vi "I2C Grove 8x8 RGB Matrix LED Examples.vi"() -> ()   [LabVIEW 2020, in "CTI-Scratchpad.lvlib"]
uses:
  CTI-Scratchpad.lvlib
  CTI/Identity.ctl
  CTI-Peripheral/RGB LED Matrix/Grove 2 RGB LED Matrix/Data Types/Colors.ctl
  CTI-Peripheral/RGB LED Matrix/Grove 2 RGB LED Matrix/Data Types/Emojis.ctl
  CTI-Peripheral/RGB LED Matrix/Grove 2 RGB LED Matrix/Data Types/Animations.ctl
  CTI/Error Reporting.ctl
  CTI/GPIO Number.ctl
  CTI/I2C Number.ctl
  CTI/Session/Session.lvclass
  CTI-Peripheral/RGB LED Matrix/Grove 2 RGB LED Matrix/Grove 2 RGB LED Matrix.lvclass
  CTI/VisaComms/VisaComms.lvclass
  CTI/CTI.lvlib
panel:
  in  "Animation":T1
  in  "Set Animation":bool
  in  "Emoji":T2 items=["smile", "laugh", "sad", "mad", "angry", "cry", "greedy", "cool", "shy", "awkward", "heart", "small heart", "broken heart", "waterdrop", "flame", "creeper", "mad creeper", "sword", "wooden sword", "crystal sword", "house", "tree", "flower", "umbrella", "rain", "monster", "crab", "duck", "rabbit", "cat", "up", "down", "left", "right", "smiley face"]
  in  "Set Emoji":bool
  in  "String":string
  in  "Set String":bool
  in  "Colour":T3 items=["red"=0, "orange"=18, "yellow"=24, "green"=82, "cyan"=127, "blue"=170, "purple"=195, "pink"=220, "white"=254, "black"=255]
  in  "Number":u16 max=9 step=1
  out "Version":string
  in  "Set Number":bool
  out "Identity":T4
  in  "stop":bool
  in  "Grove Connector":enum16{"I2C0", "I2C1"}(ring)
  out "error out":errorcluster
  in  "Port":refnum<visa-resource-name>="COM4"
  # "https://wiki.seeedstudio.com/Grove-RGB_LED_Matrix_w-Driver/"
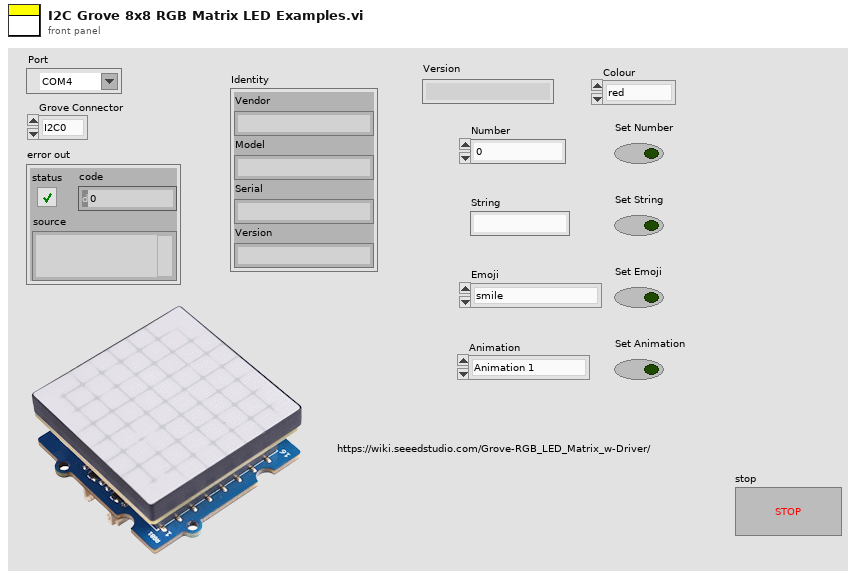
[diagram p1: front panel]
types:
  T1 = typedef "CTI-Peripheral.lvlib/Grove 2 RGB LED Matrix.lvclass/Animations.ctl" = enum16{"Animation 1", "Animation 2", "Rainbow Cycle", "Fire", "Walking", "Broken Heart"}
  T2 = typedef "CTI-Peripheral.lvlib/Grove 2 RGB LED Matrix.lvclass/Emojis.ctl" = u16
  T3 = typedef "CTI-Peripheral.lvlib/Grove 2 RGB LED Matrix.lvclass/Colors.ctl" = u8
  T4 = typedef "CTI.lvlib/Identity.ctl" = cluster{"Vendor":string, "Model":string, "Serial":string, "Version":string}
  T5 = typedef "CTI.lvlib/Error Reporting.ctl" = enum16{"Minimal", "Moderate", "Full"}
  T6 = typedef "CTI.lvlib/I2C Number.ctl" = i8
  T7 = typedef "CTI.lvlib/GPIO Number.ctl" = i8
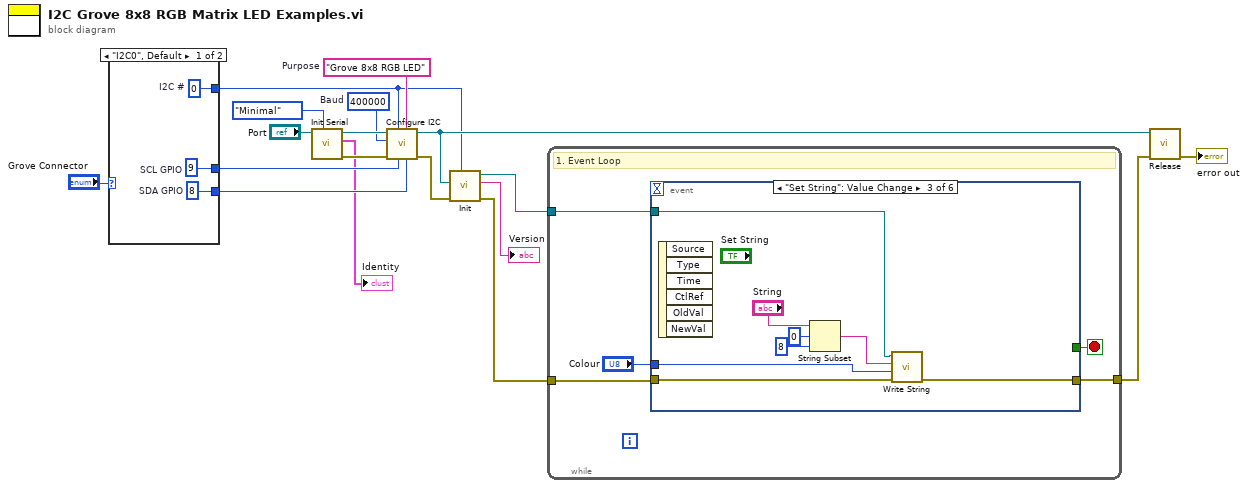
[diagram p0: block diagram]
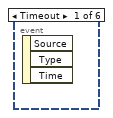
[diagram p2: hidden frame]
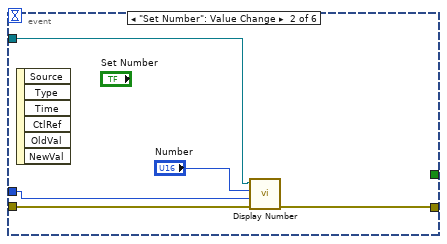
[diagram p3: hidden frame]
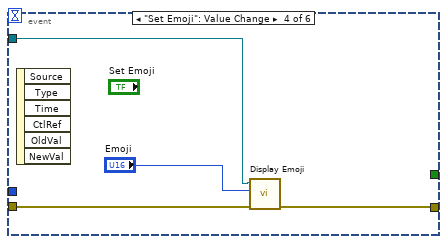
[diagram p4: hidden frame]
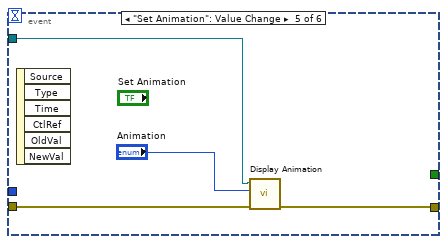
[diagram p5: hidden frame]
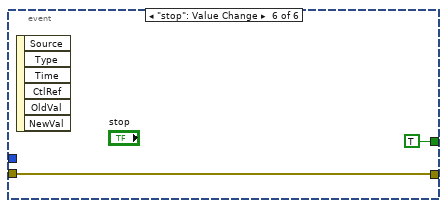
[diagram p6: hidden frame]
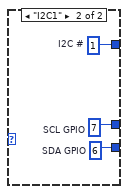
[diagram p7: hidden frame]
diagram:
  w13 = "Grove 8x8 RGB LED"  # Purpose
  w14 = u32 400000  # Baud
  n1 = case shown="\"I2C0\", Default" "Grove Connector" {
    tunnel: [w21 w24] -> w9
    tunnel: [w20 w23] -> w8
    tunnel: [w19 w22] -> w7
    frame "I2C0", Default {
      w19 = T6 0  # I2C #
      w20 = T7 8  # SDA GPIO
      w21 = T7 9  # SCL GPIO
    }
    frame "I2C1" {
      w22 = T6 1  # I2C #
      w23 = T7 6  # SDA GPIO
      w24 = T7 7  # SCL GPIO
    }
  }
  n2 = call "Init Serial.vi"("Error Checking (Full)"=Error_Reporting."Minimal", "VISA resource name in"="Port") -> ("error out"=w15:errorcluster, "Identity"=→"Identity":T4, "Session"=w16:refnum<class "Session.lvclass">)  [unwired: 7 in]
  n3 = call "Configure I2C.vi"("SDA GPIO"=w8, "Purpose (\"I2C\")"=w13, "SCL GPIO"=w9, "I2C #"=w7, "error in (no error)"=w15, "Baud"=w14, "Session in"=w16) -> ("error out"=w12:errorcluster, "Session out"=w11:refnum<class "Session.lvclass">)  [unwired: 3 in]
  n4 = call "Init.vi"("I2C #"=w7, "error in (no error)"=w12, "Session In"=w11) -> ("error out"=w5:errorcluster, "Version"=→"Version":string, "Grove 2 RGB LED Matrix Out"=w2:refnum<class "Grove 2 RGB LED Matrix.lvclass">)  [unwired: 6 in]
  n5 = while {
    tunnel: w5 -> [w28]
    tunnel: [w27] -> w4
    tunnel: w2 -> [w29]
    stop <- w26 stop-if-true
    # "1. Event Loop"
    n6 = event shown="[2] \"Set String\": Value Change" {
      selector: _ -> [_ _ _ _ _ _]
      dyn-events: _ -> [_ _ _ _ _ _]
      timeout: _ -> [_ _ _ _ _ _]
      tunnel: w29 -> [_ w32 w40 w44 w48 _]
      tunnel: w28 -> [_ w34 w42 w46 w50 w52]
      tunnel: [_ w33 w41 w45 w49 w52] -> w27
      tunnel: [_ _ _ _ _ TRUE] -> w26
      tunnel: "Colour" -> [_ w30 w39 _ _ _]
      event Timeout {
        n7 = event-data() -> ()  [unwired: 1 in, 3 out]
      }
      event "Set Number": Value Change {
        n8 = event-data() -> ()  [unwired: 1 in, 6 out]
        n9 = call-dynamic "Display Number.vi"("error in (no error)"=w34, "Colour"=w30, "Numeric"="Number", "Grove 2 RGB LED Matrix In"=w32) -> ("error out"=w33:errorcluster)  [unwired: 6 in, 1 out]
      }
      event "Set String": Value Change {
        n10 = event-data() -> ()  [unwired: 1 in, 6 out]
        n11 = String Subset(string="String", offset (0)=0, length (rest)=8 ("length (rest)")) -> (substring=w35:string)
        n12 = call-dynamic "Write String.vi"("error in (no error)"=w42, "Colour"=w39, "String"=w35, "Grove 2 RGB LED Matrix In"=w40) -> ("error out"=w41:errorcluster)  [unwired: 6 in, 1 out]
      }
      event "Set Emoji": Value Change {
        n13 = event-data() -> ()  [unwired: 1 in, 6 out]
        n14 = call-dynamic "Display Emoji.vi"("error in (no error)"=w46, "Emoji"="Emoji", "Grove 2 RGB LED Matrix In"=w44) -> ("error out"=w45:errorcluster)  [unwired: 7 in, 1 out]
      }
      event "Set Animation": Value Change {
        n15 = event-data() -> ()  [unwired: 1 in, 6 out]
        n16 = call-dynamic "Display Animation.vi"("error in (no error)"=w50, "Animations"="Animation", "Grove 2 RGB LED Matrix In"=w48) -> ("error out"=w49:errorcluster)  [unwired: 7 in, 1 out]
      }
      event "stop": Value Change {
        n17 = event-data() -> ()  [unwired: 1 in, 6 out]
      }
    }
  }
  n18 = call-dynamic "Release.vi"("error in (no error)"=w4, "Session in"=w11) -> ("error out"=→"error out":errorcluster)  [unwired: 9 in]
